vi "_PC_Pub_FM ctrlTempStateMachine.vi"(5 "pause? (F)":bool=TRUE, 7 "function":T1(ring), 8 "error in (no error)":errorcluster, 10 "sourceData":waveform(sgl)) -> (0 "error out":errorcluster, 1 "finish? (F)":bool, 2 "outputData":waveform(sgl))   [LabVIEW 2018]
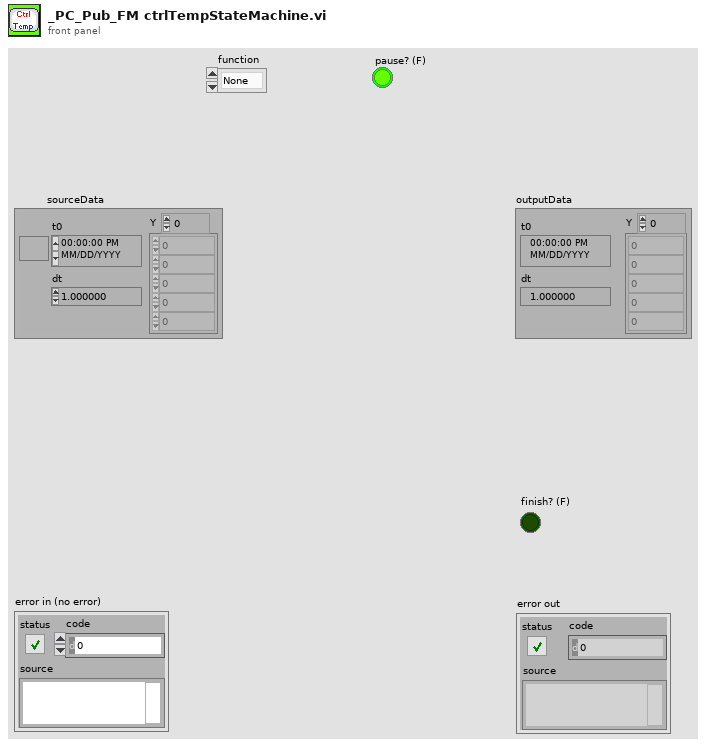
[diagram p1: front panel]
types:
  T1 = enum16{"None", "Init", "Write", "Read", "PauseRead", "FinishCheck"}
  T2 = enum16{"open", "replace", "create", "open or create", "replace or create", "replace or create with confirmation"}
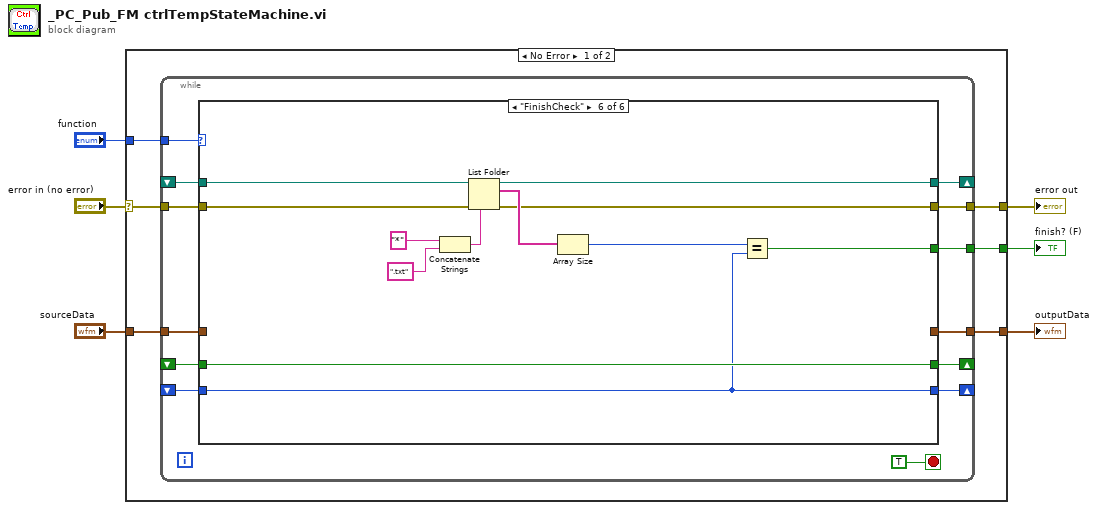
[diagram p0: block diagram]
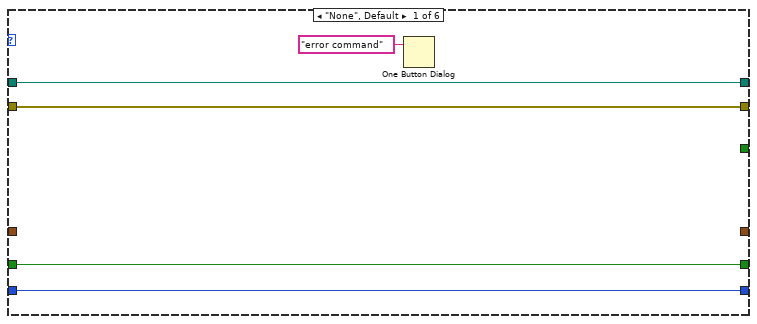
[diagram p2: hidden frame]
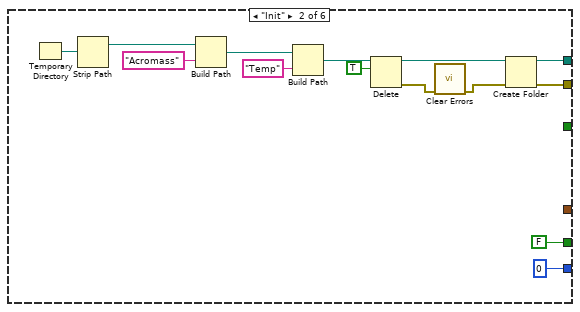
[diagram p3: hidden frame]
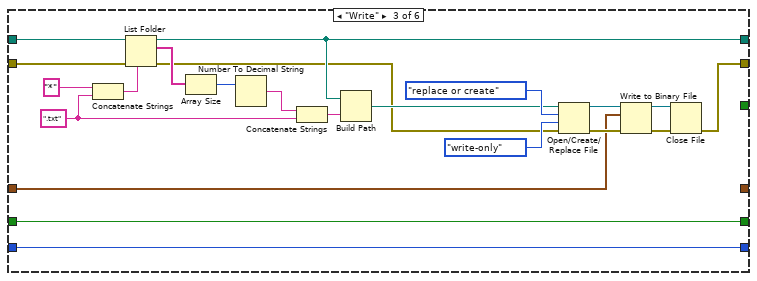
[diagram p4: hidden frame]
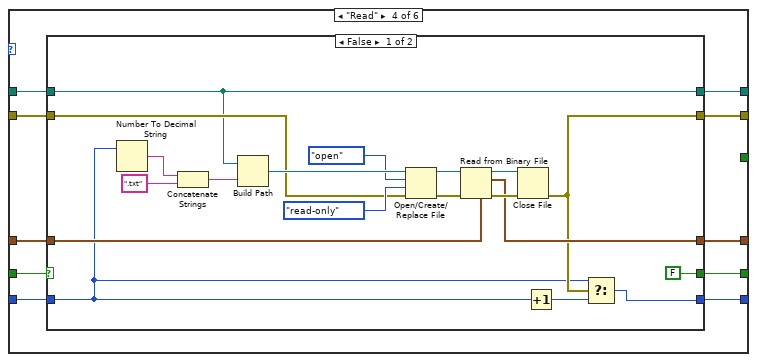
[diagram p5: hidden frame]
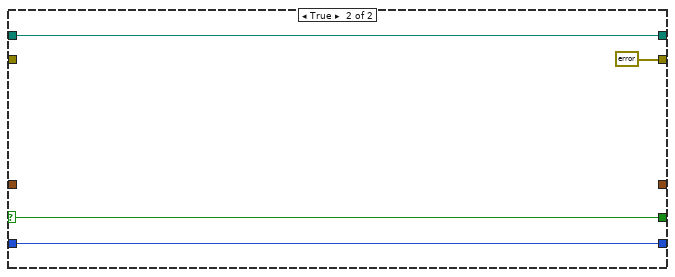
[diagram p6: hidden frame]
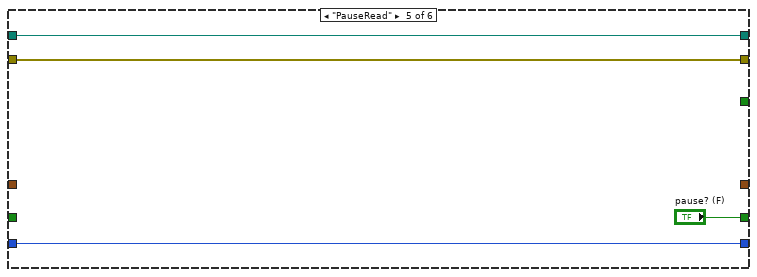
[diagram p7: hidden frame]
diagram:
  n1 = case shown="No Error" "error in (no error)" {
    selector: "error in (no error)" -> [w9 w116]
    tunnel: "function" -> [w12 _]
    tunnel: "sourceData" -> [w11 _]
    tunnel: [w10 _] -> w4
    tunnel: [w8 w116] -> w2
    tunnel: [w7 _] -> w1
    frame No Error {
      n2 = while {
        tunnel: w12 -> [w25]
        shift-right: [w24] -> _
        shift-left: _ -> [w21]
        tunnel: w11 -> [w23]
        tunnel: [w22] -> w10
        tunnel: w9 -> [w20]
        tunnel: [w19] -> w8
        shift-right: [w16] -> _
        shift-left: _ -> [w18]
        shift-right: [w15] -> _
        shift-left: _ -> [w14]
        tunnel: [w13] -> w7
        stop <- TRUE stop-if-true
        n3 = case shown="\"FinishCheck\"" w25 {
          tunnel: [w30 w34 w58 w67 w102 w110] -> w24
          tunnel: w23 -> [_ _ w50 w74 _ _]
          tunnel: [_ _ _ w73 _ _] -> w22
          tunnel: w21 -> [w30 _ w66 w76 w102 w111]
          tunnel: w20 -> [w28 _ w65 w75 w101 w109]
          tunnel: [w28 w33 w47 w72 w101 w106] -> w19
          tunnel: w18 -> [w27 _ w46 w70 w100 w107]
          tunnel: [w27 u64 0 w46 w71 w100 w107] -> w16
          tunnel: [w26 FALSE ("stop? (F)") w45 w68 "pause? (F)" w108] -> w15
          tunnel: w14 -> [w26 _ w45 w69 _ w108]
          tunnel: [_ _ _ _ _ w105] -> w13
          frame "None", Default {
            n4 = One Button Dialog(message="error command") -> ()  [unwired: 1 in, 1 out]
          }
          frame "Init" {
            n5 = Temporary Directory() -> (w42:path)
            n6 = Strip Path(path=w42) -> (stripped path=w44:path)  [unwired: 1 out]
            n7 = Build Path(base path=w44, name or relative path="Acromass") -> (appended path=w41:path)
            n8 = Build Path(base path=w41, name or relative path="Temp") -> (appended path=w39:path)
            n9 = Delete(path (use dialog)=w39, entire hierarchy (F)=TRUE) -> (deleted path=w37:path, error out=w36:errorcluster)  [unwired: 3 in, 1 out]
            n10 = call <vilib>:"Clear Errors.vi"("error in (no error)"=w36) -> ("error out"=w35:errorcluster)  [unwired: 5 in, 1 out]
            n11 = Create Folder(path (use dialog)=w37, error in=w35) -> (created path=w34:path, error out=w33:errorcluster)  [unwired: 1 in, 1 out]
          }
          frame "Write" {
            w59 = ".txt"
            n12 = Concatenate Strings("*" ("string"), w59) -> (w60:string)
            n13 = List Folder(path=w66, pattern=w60, error in=w65) -> (path out=w58:path, filenames=w64:string[], error out=w53:errorcluster)  [unwired: 1 in, 1 out]
            n14 = Array Size(array=w64) -> (size(s)=w63:i32)
            n15 = Number To Decimal String(number=w63) -> (decimal integer string=w62:string)  [unwired: 1 in]
            n16 = Concatenate Strings(w62, w59) -> (w57:string)
            n17 = Build Path(base path=w58, name or relative path=w57) -> (appended path=w54:path)
            n18 = Open/Create/Replace File(file path (use dialog)=w54, error in=w53, operation (0:open)=T2."replace or create", access (0:read/write)=enum16{"read/write", "read-only", "write-only"}."write-only") -> (refnum out=w52:refnum<file>, error out=w51:errorcluster)  [unwired: 2 in, 1 out]
            n19 = Write to Binary File(file (use dialog)=w52, data=w50, error in=w51) -> (refnum out=w49:refnum<file>, error out=w48:errorcluster)  [unwired: 3 in, 1 out]
            n20 = Close File(refnum=w49, error in=w48) -> (error out=w47:errorcluster)  [unwired: 1 out]
          }
          frame "Read" {
            n21 = case shown="False" w69 {
              selector: w69 -> [_ w98]
              tunnel: w76 -> [w77 w99]
              tunnel: w75 -> [w85 _]
              tunnel: w74 -> [w84 _]
              tunnel: [w83 _] -> w73
              tunnel: [w82 errorcluster {"status"=TRUE, "code"=6999, "source"="Pause Read"} ("error out")] -> w72
              tunnel: [w80 w97] -> w71
              tunnel: w70 -> [w79 w97]
              tunnel: [FALSE w98] -> w68
              tunnel: [w77 w99] -> w67
              frame False {
                n22 = Number To Decimal String(number=w79) -> (decimal integer string=w93:string)  [unwired: 1 in]
                n23 = Concatenate Strings(w93, ".txt") -> (w94:string)
                n24 = Build Path(base path=w77, name or relative path=w94) -> (appended path=w88:path)
                n25 = Open/Create/Replace File(file path (use dialog)=w88, error in=w85, operation (0:open)=T2."open", access (0:read/write)=enum16{"read/write", "read-only", "write-only"}."read-only") -> (refnum out=w92:refnum<file>, error out=w91:errorcluster)  [unwired: 2 in, 1 out]
                n26 = Read from Binary File(5:w84, 8:w91, 11:w92) -> (0:w89:errorcluster, 2:w83:waveform(sgl), 3:w90:refnum<file>)  [unwired: 3 in, 1 out]
                n27 = Close File(refnum=w90, error in=w89) -> (error out=w82:errorcluster)  [unwired: 1 out]
                n28 = Increment(x=w79) -> (x+1=w81:u64)
                n29 = Select(t=w79, s=w82, f=w81) -> (s? t:f=w80:u64)
              }
              frame True {
              }
            }
          }
          frame "PauseRead" {
          }
          frame "FinishCheck" {
            n30 = Concatenate Strings("*" ("string"), ".txt") -> (w113:string)
            n31 = List Folder(path=w111, pattern=w113, error in=w109) -> (path out=w110:path, filenames=w115:string[], error out=w106:errorcluster)  [unwired: 1 in, 1 out]
            n32 = Array Size(array=w115) -> (size(s)=w104:i32)
            n33 = Equal?(x=w104, y=w107) -> (x = y?=w105:bool)
          }
        }
      }
    }
    frame Error {
    }
  }
  "outputData" <- w4
  "error out" <- w2
  "finish? (F)" <- w1
